vi "SQL_QueryReturn.vi"(9 "SQL query":string, 11 "ConnectionDSN":string) -> (1 "data":string[][](array[string]))   [LabVIEW 2017]
uses:
  <vilib>/addons/database/Connection.llb/DB Tools Open Connec (String).vi
  <vilib>/addons/database/Connection.llb/Conn Execute.vi
  <vilib>/addons/database/Recordset.llb/Rec Fetch Recordset Data (R).vi
  <vilib>/addons/database/_DB Variant To Data/Database Variant To Data.xnode
  <vilib>/addons/database/NI_Database_API.lvlib
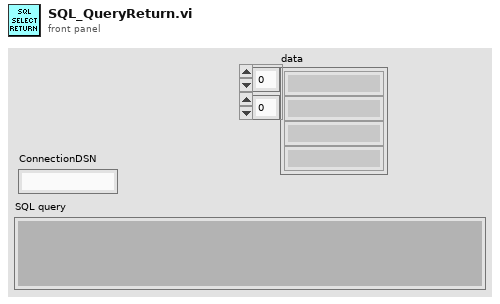
[diagram p1: front panel]
types:
  T1 = typedef "NI_Database_API.lvlib/Conn ObjectReference.ctl" = refnum<k1>
  T2 = typedef "NI_Database_API.lvlib/Rec ObjectReference.ctl" = refnum<k1>
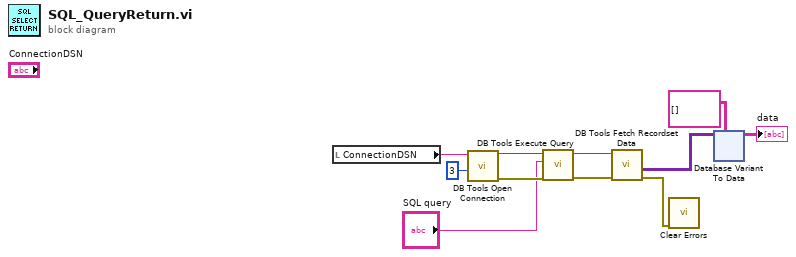
[diagram p0: block diagram]
diagram:
  n1 = local read "ConnectionDSN"() -> (w11:string)
  n2 = call-poly <vilib>:"DB Tools Open Connection.vi"("connection timeout (15)"=3, "connection information"=w11) -> ("error out"=w8:errorcluster, "connection reference"=w10:T1)  [unwired: 6 in]
  n3 = call-poly <vilib>:"DB Tools Execute Query.vi"("error in (no error)"=w8, "SQL query"="SQL query", "connection reference"=w10) -> ("error out"=w7:errorcluster, "recordset reference"=w9:T2)  [unwired: 5 in]
  n4 = call-poly <vilib>:"DB Tools Fetch Recordset Data.vi"("error in (no error)"=w7, "recordset reference"=w9) -> ("error out"=w1:errorcluster, "recordset data"=w5:variant[][])  [unwired: 3 in, 1 out]
  n5 = call <vilib>:"Clear Errors.vi"("error in (no error)"=w1) -> ()  [unwired: 5 in, 2 out]
  n6 = xnode "Database Variant To Data"("database variant"=w5, "type"=string[][] []) -> ("data"=→"data":string[][])  [unwired: 1 in, 1 out]
